vi "Append to average (subVi).vi"(1 "Array in":dbl[][](array[numeric]), 2 "Average array":dbl[][](array[numeric])) -> (0 "Average array out":dbl[][](array[numeric]))   [LabVIEW 2016]
panel:
  out "previous value":dbl
  out "value to add":dbl
  out "mass to add":dbl
  out "number":dbl
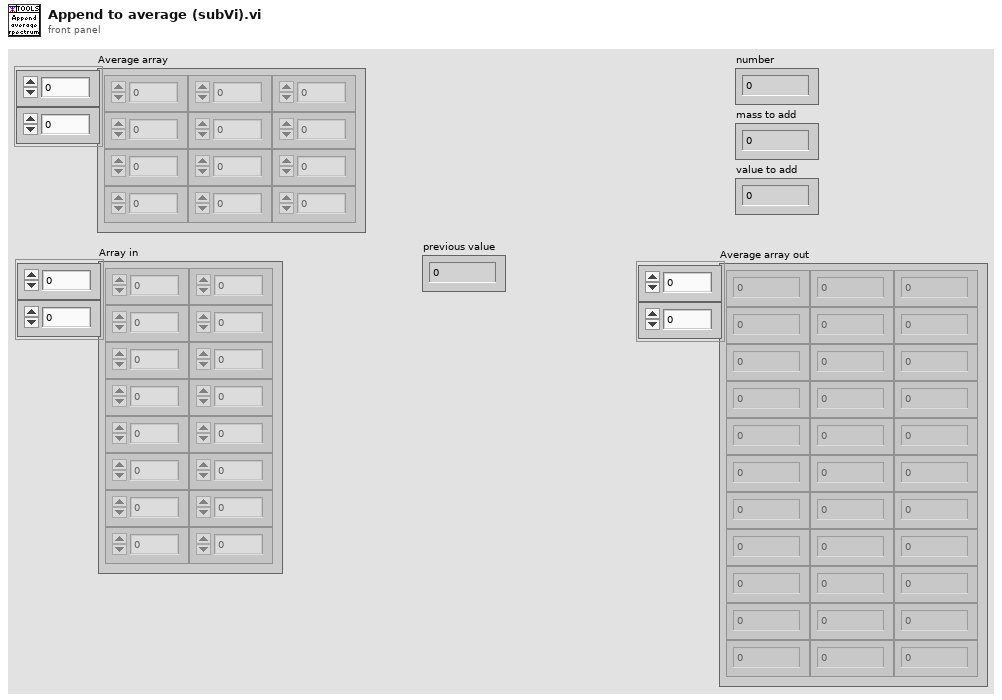
[diagram p1: front panel]
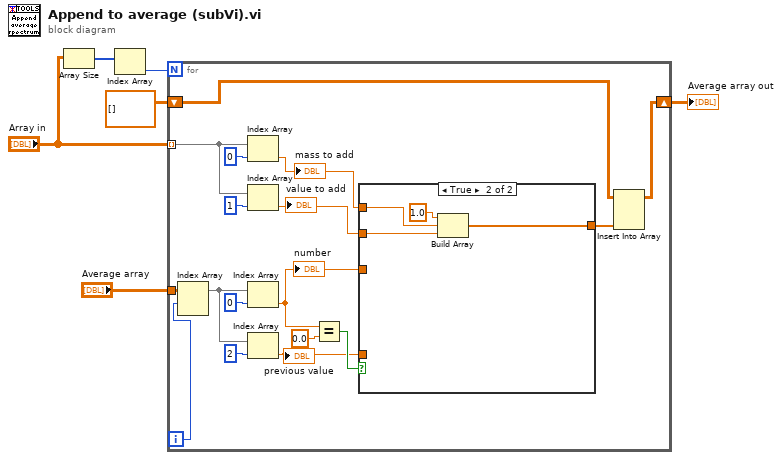
[diagram p0: block diagram]
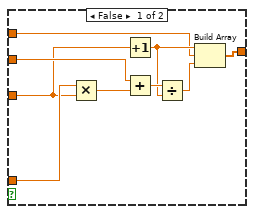
[diagram p2: hidden frame]
diagram:
  n1 = Array Size(array="Array in") -> (size(s)=w6:i32[])
  n2 = Index Array(array=w6) -> (element=w5:i32)  [unwired: 1 in]
  n3 = for {
    N: w5 -> [_]
    tunnel: "Array in" -> [w15] mode=indexing
    tunnel: "Average array" -> [w21]
    shift-right: [w12] -> w1
    shift-left: dbl[][] [] ("Average array") -> [w10]
    i -> [w7]
    n4 = Index Array(array=w21, index (row)=w7) -> (element=w8:dbl[])  [unwired: 1 in]
    n5 = Index Array(array=w15, index=0) -> (element=w14:dbl)
    "mass to add" <- w14
    n6 = Index Array(array=w15, index=1) -> (element=w13:dbl)
    "value to add" <- w13
    n7 = Index Array(array=w8, index=0) -> (element=w17:dbl)
    "number" <- w17
    n8 = Index Array(array=w8, index=2) -> (element=w11:dbl)
    "previous value" <- w11
    n9 = Equal?(x=w17, y=0.0) -> (x = y?=w19:bool)
    n10 = case shown="True" w19 {
      tunnel: w17 -> [w28 _]
      tunnel: w14 -> [w26 w36]
      tunnel: w13 -> [w30 w35]
      tunnel: [w24 w34] -> w9
      tunnel: w11 -> [w32 _]
      frame False {
        n11 = Multiply(x=w32, y=w28) -> (x*y=w31:dbl)
        n12 = Increment(x=w28) -> (x+1=w27:dbl)
        n13 = Add(x=w30, y=w31) -> (x+y=w29:dbl)
        n14 = Divide(x=w29, y=w27) -> (x/y=w25:dbl)
        n15 = Build Array(w27, w26, w25) -> (w24:dbl[])
      }
      frame True {
        n16 = Build Array(1.0, w36, w35) -> (w34:dbl[])
      }
    }
    n17 = Insert Into Array(array=w10, new element=w9) -> (w12:dbl[][])  [unwired: 2 in]
  }
  "Average array out" <- w1
